vi "To Wheel Angle.vi"(2 "error in (no error)":errorcluster, 3 "Servo PWM":dbl, 4 "Car.lvclass":refnum<class "Car.lvclass">) -> (0 "error out":errorcluster, 1 "Wheel Angle":dbl)   [LabVIEW 2015, in "Car.lvclass"]
uses:
  Car.lvclass
  Car.lvclass/Car.ctl
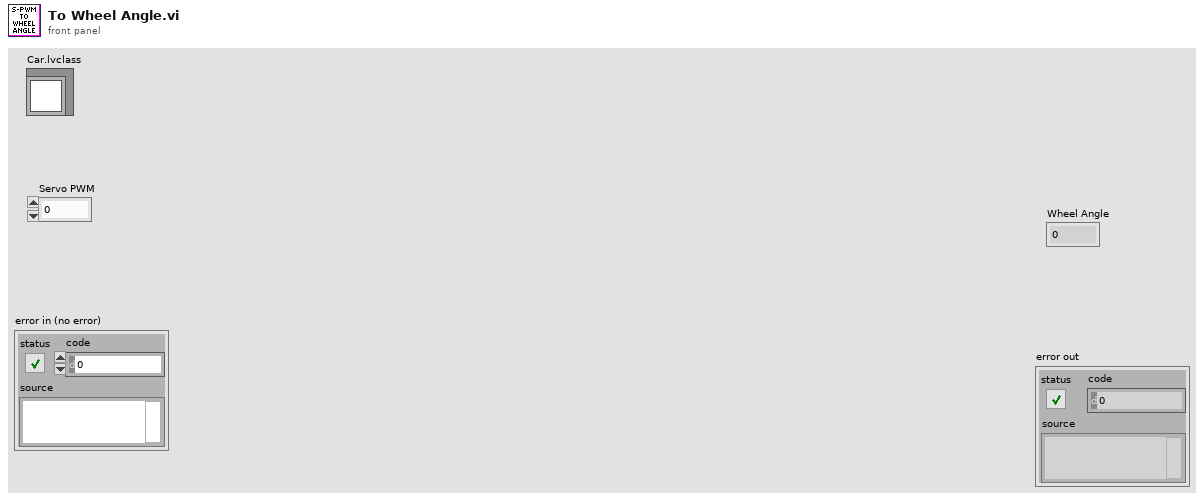
[diagram p1: front panel]
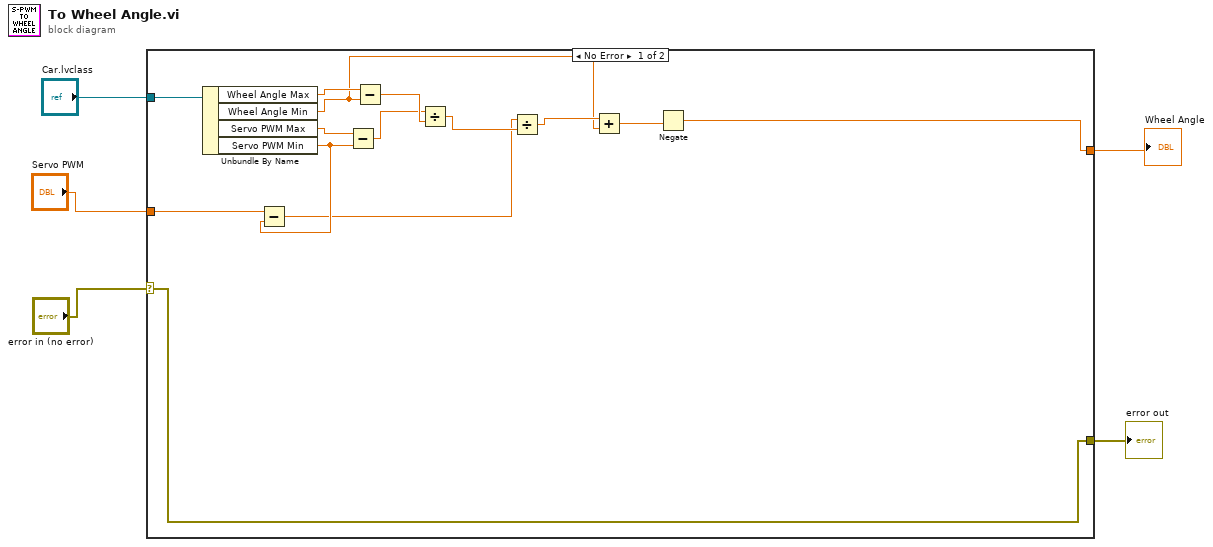
[diagram p0: block diagram]
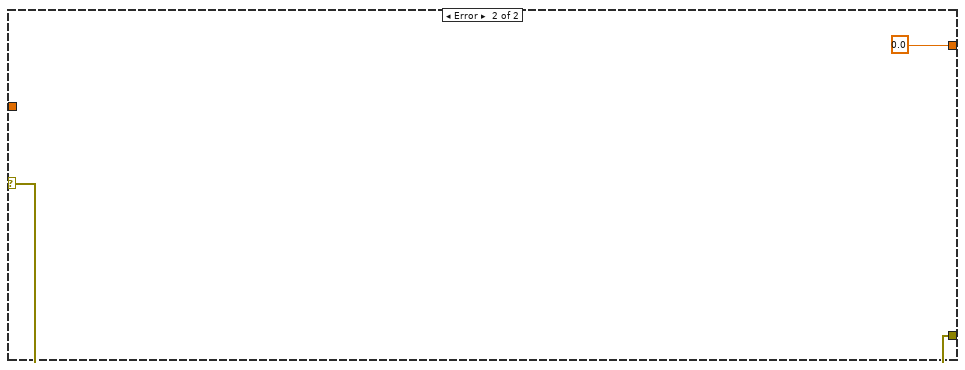
[diagram p2: hidden frame]
diagram:
  n1 = case shown="No Error" "error in (no error)" {
    selector: "error in (no error)" -> [w19 w20]
    tunnel: [w19 w20] -> w4
    tunnel: [w6 0.0] -> w3
    tunnel: "Car.lvclass" -> [w18 _]
    tunnel: "Servo PWM" -> [w13 _]
    frame No Error {
      n2 = Unbundle By Name(w18) -> ("Wheel Angle Max"=w17:dbl, "Wheel Angle Min"=w8:dbl, "Servo PWM Max"=w16:dbl, "Servo PWM Min"=w12:dbl)
      n3 = Subtract(x=w13, y=w12) -> (x-y=w10:dbl)
      n4 = Subtract(x=w16, y=w12) -> (x-y=w14:dbl)
      n5 = Subtract(x=w17, y=w8) -> (x-y=w15:dbl)
      n6 = Divide(x=w14, y=w15) -> (x/y=w11:dbl)
      n7 = Divide(x=w10, y=w11) -> (x/y=w9:dbl)
      n8 = Add(x=w9, y=w8) -> (x+y=w7:dbl)
      n9 = Negate(x=w7) -> (-x=w6:dbl)
    }
    frame Error {
    }
  }
  "error out" <- w4
  "Wheel Angle" <- w3
